vi "noisysinewave.vi"() -> (0 "x+y":waveform(dbl))   [LabVIEW 2016]
uses:
  <vilib>/measure/NI_MABase.lvlib
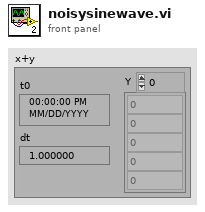
[diagram p1: front panel]
types:
  T1 = enum16{"Sine Wave", "Triangle Wave", "Square Wave", "Sawtooth Wave"}
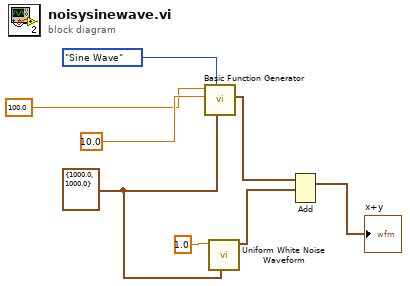
[diagram p0: block diagram]
diagram:
  w6 = cluster{"Fs":dbl, "#s":dbl} {"Fs"=1000.0, "#s"=1000.0} ("sampling info")
  n1 = call <vilib>:"Basic Function Generator.vi"("sampling info"=w6, "signal type"=T1."Sine Wave", "amplitude"=10.0, "frequency"=100.0) -> ("signal out"=w7:waveform(dbl))  [unwired: 5 in, 2 out]
  n2 = call <vilib>:"Uniform White Noise Waveform.vi"("sampling info"=w6, "amplitude"=1.0) -> ("signal out"=w8:waveform(dbl))  [unwired: 8 in, 1 out]
  n3 = Add(1:w8, 2:w7) -> (0:→"x+y":waveform(dbl))  [unwired: 1 in, 1 out]
